vi "Dashboard Main.vi"() -> ()   [LabVIEW 2014]
uses:
  <vilib>/event_ctls.llb/eventvkey.ctl
  <vilib>/Rock Robotics/WPI/Dashboard/WPI_DashboardLogging Global.vi
  <vilib>/Rock Robotics/Network Tables/SD Read String Array.vi
  <vilib>/Rock Robotics/Network Tables/SD Read String.vi
  <vilib>/Utility/config.llb/Write Key (String).vi
  <vilib>/Utility/config.llb/Write Key (I32).vi
  <vilib>/Utility/cursorutil.llb/Set Cursor (Icon Pict).vi
  <vilib>/Utility/config.llb/NI_LVConfig.lvlib
panel:
  out "path":path
  in  "CameraView":bool
  in  "TCP":refnum<k5>
  in  "Rec Mode":enum32{"Stop", "Record", "Playback"}(radio)
  in  "Vision":u16(ring) items=["Camera Off", "USB Camera SW", "USB Camera HW", "IP Camera"]
  out "Camera IP":string
  out "Image Message":string="Timeout in Camera Communications"
  in  "Dashboard Tab":T1(tab)
  in  "Camera Settings":T2={"Frame Rate"=30, "Compression"=30, "Size"=1} {"Frame Rate" scale=1.0..30.0; "Size" items=["640x480", "320x240", "160x120"]}
  out "MotorChart R":cluster{"Numeric":dbl, "Numeric":dbl}(graph)
  out "MotorChart L":T3(graph)
  out "MotorSliders R":cluster{"MotorSlide1":dbl, "MotorSlide2":dbl} {"MotorSlide2" scale=-1.0..1.0 scale format="%#_2e"; "MotorSlide1" scale=-1.0..1.0 scale format="%#_2e"}
  out "MotorSliders L":T4 {"MotorSlide4 2" scale=0.0..14.0 scale format="%#_2e"; "MotorSlide2" scale=-1.0..1.0 scale format="%#_2e"; "MotorSlide1" scale=-1.0..1.0 scale format="%#_2e"}
  out "Gyro":dbl(knob) scale=0.0..360.0
  out "JS1 Z":dbl(slide) scale=-1.0..1.0 scale format="%#_2e"
  out "JS1 Graph":cluster{"X":dbl, "Y":dbl}[](graph)
  out "JS1 Buttons":T5
  out "JS2 Z":dbl(slide) scale=-1.0..1.0 scale format="%#_2e"
  out "JS2 Graph":cluster{"X":dbl, "Y":dbl}[](graph)
  out "JS2 Buttons":T5
  out "Mode":T6(ring)=enum."Auto Disabled"
  in  "DB Camera Config":bool
  out "fps":dbl format="%#.1g"
  out "Mbps":dbl format="%#.1g"
  out "Mbps 2":bool
  in  "DB/String 9":string
  in  "DB/String 8":string
  in  "DB/String 7":string
  in  "DB/String 6":string
  in  "DB/String 5":string
  in  "DB/String 4":string
  in  "DB/String 3":string
  in  "DB/String 2":string
  in  "DB/String 1":string
  in  "DB/String 0":string
  in  "DB/Slider 0":dbl(slide) scale=0.0..5.0
  in  "DB/Slider 1":dbl(slide) scale=0.0..5.0
  in  "DB/Slider 2":dbl(slide) scale=0.0..5.0
  in  "DB/Slider 3":dbl(slide) scale=0.0..5.0
  out "DB/LED 3":bool
  out "DB/LED 2":bool
  out "DB/LED 1":bool
  out "DB/LED 0":bool
  in  "DB/Button 3":bool
  in  "DB/Button 2":bool
  in  "DB/Button 1":bool
  in  "DB/Button 0":bool caption="New Name"
  out "Command":string
  in  "Enable Scripting":bool
  in  "Save":bool
  in  "Auton Edit Area":string
  in  "Edit":bool
  in  "Auton List":string(combo)
  out "CMD":string
  in  "Test Slider":dbl(slide) scale=0.0..100.0 scale format="%#_3g"
  in  "On/Off":bool caption="Solenoid"
  in  "Test Name":u16(ring) items=["Select the test to run...", "Example Test", "-------------------------------", "List of tests is built in robot code.", "Replace with your own automated tests."]
  in  "Test Tree":string(tree)
  in  "Motor":cluster{"Value":dbl, "Enable":bool} {"Value" scale=-1.0..1.0 scale format="%#_3g"}
  out "Progress":T7 {"Test Progress" scale=0.0..100.0}
  in  "Rev/Fwd":cluster{"Forward":bool, "Reverse":bool}
  in  "Test Ring":u16(ring) items=["Monochrome", "Color"]
  in  "Listbox":i32(listbox)
  out "Tree":string(tree)
  out "Camera Image":T8(plugin-control)
  out "Boolean":bool
  # "Left"
  # "Front"
  # "Right"
  # "Battery"
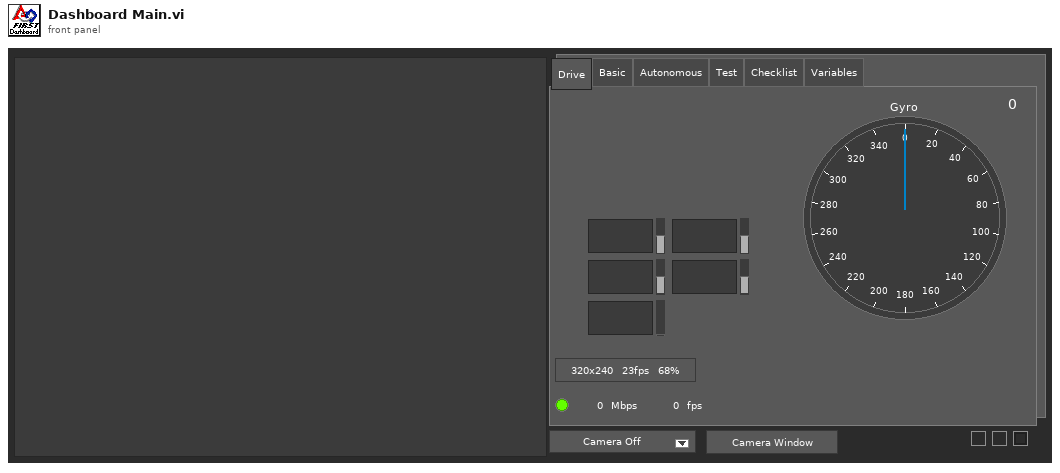
[diagram p1: front panel]
types:
  T1 = enum32{"Drive", "Basic", "Autonomous", "Test", "Checklist", "Variables"}
  T2 = cluster{"Frame Rate":i32, "Compression":i32, "Size":u16}
  T3 = cluster{"Numeric":dbl, "Numeric":dbl, "Battery V":dbl}
  T4 = cluster{"MotorSlide1":dbl, "MotorSlide2":dbl, "MotorSlide4 2":dbl}
  T5 = cluster{bool, bool, bool, bool, bool, bool, bool, bool, bool, bool, bool, bool}
  T6 = enum8{"Tele-Op Disabled", "Tele-Op Enabled", "Auto Disabled", "Auto Enabled", "Test Disabled", "Test Enabled", "Disconnected", "No Code", "E-Stop"}
  T7 = cluster{"Test Progress":u8, "Test Progress Text":string}
  T8 = typedef "IMAQ Image.ctl" = refnum<image>
  T9 = enum32{"Drive", "Basic", "Custom", "Test", "Checklist", "Variables"}
  T10 = typedef "Image Type" = u32
  T11 = cluster{"Camera Image":refnum<vi>, "Dashboard Tab":refnum<vi>, "Boolean":refnum<vi>, "Vision":refnum<vi>, "Rec Mode":refnum<vi>, "Test Slider":refnum<vi>, "On/Off ":refnum<vi>, "Test Ring":refnum<vi>, "Rev/Fwd":refnum<vi>, "Test Name":refnum<vi>, "Motor":refnum<vi>, "Progress":refnum<vi>, "CheckList":refnum<vi>, "Tree":refnum<vi>, "Test Tree":refnum<vi>}
  T12 = cluster{"Error Strings":string, "Disable Counts":cluster{u16, u16}, "Rail Faults":cluster{u16, u16, u16}, "Robot IP":string, "DB Mode":u8, "Event Info":cluster{"Name":string, "Type":u8, "Number":u16, "Replay":u8}, "Camera Addr":string}
  T13 = cluster{"Storage":cluster{"Disk Free":u64, "RAM Block":u32, "RAM free":u32}, "CPU Utilization":cluster{"CPU % ISR":sgl, "CPU % Time Crit":sgl, "CPU % Timed Str":sgl, "CPU % High":sgl, "CPU % Above":sgl, "CPU % Normal":sgl, "CPU % Low":sgl}, "CAN":cluster{"% Bus Utilization":sgl, "Bus Off Cnt":u32, "TX_FIFO Full Cnt":u32, "Receive Error Cnt":u8, "Transmit Error Cnt":u8}, "HID":cluster{"HID Outputs":u32, "Rumble Low":u16, "Rumble High":u16}[]}
  T14 = cluster{"Status bits":cluster{"Test Mode":bool, "Autonomous":bool, "Enabled":bool, "Code Start":bool, "Brownout":bool, "Reserved 2":bool, "Reserved 3":bool, "E-Stop":bool}, "Code Trace":cluster{"Disabled":bool, "TeleOp":bool, "Auto":bool, "Test":bool}, "Controller Type":enum16{"unknown", "cRIO", "roboRio"}, "Code?":enum16{"unknown", "noCode", "code"}, "Battery V":dbl}
  T15 = cluster{"Control Bits":cluster{"TestMode":bool, "Autonomous":bool, "Enabled":bool, "FMS Present":bool, bool, bool, bool, "E-Stop":bool}, "Team Station ":u8, "Countdown":sgl, "Joystick Values":cluster{"Axes":dbl[], "Buttons":bool[], "POVs":i16[]}[]}
  T16 = cluster{"Axes":dbl[], "Buttons":bool[], "POVs":i16[]}[]
  T17 = cluster{"Axes":dbl[], "Buttons":bool[], "POVs":i16[]}
  T18 = cluster{"Buttons[0]":bool, "Buttons[1]":bool, "Buttons[2]":bool, "Buttons[3]":bool, "Buttons[4]":bool, "Buttons[5]":bool, "Buttons[6]":bool, "Buttons[7]":bool, "Buttons[8]":bool, "Buttons[9]":bool, "Buttons[10]":bool, "Buttons[11]":bool}
  T19 = typedef "NI_LVConfig.lvlib/Config Data RefNum.ctl" = refnum<k1>
  T20 = cluster{"Operation":enum16{"Update", "Clear"}, "Color Box":u32}[]
  T21 = typedef "eventvkey.ctl" = enum16{"ASCII", "Enter", "Return", "Shift", "Ctrl", "Alt", "Cmd", "Opt", "Caps", "NumLock", "Clear", "Break", "Up", "Down", "Left", "Right", "Insert", "Delete", "Home", "End", "PageUp", "PageDown", "Escape", "Help", "Pause", "ScrollLock", "F1", "F2", "F3", "F4", "F5", "F6", "F7", "F8", "F9", "F10", "F11", "F12", "F13", "F14", "F15", "F16", "F17", "F18", "F19", "F20", "F21", "F22", "F23", "F24", "Play", "VolumeUp", "VolumeDown", "Mute", "Two Byte Char"}
  T22 = cluster{"Image Size":bool, "Image Type":bool, "Pixel Value":bool, "ROI Information":bool, "Zoom Factor":bool}
  T23 = enum8{"Enabled", "Disabled", "Disabled and Grayed Out"}
  T24 = enum16{"open", "replace", "create", "open or create", "replace or create", "replace or create with confirmation"}
  T25 = cluster{"Operation":enum16{"Update", "Clear"}, "Color Box":u32}
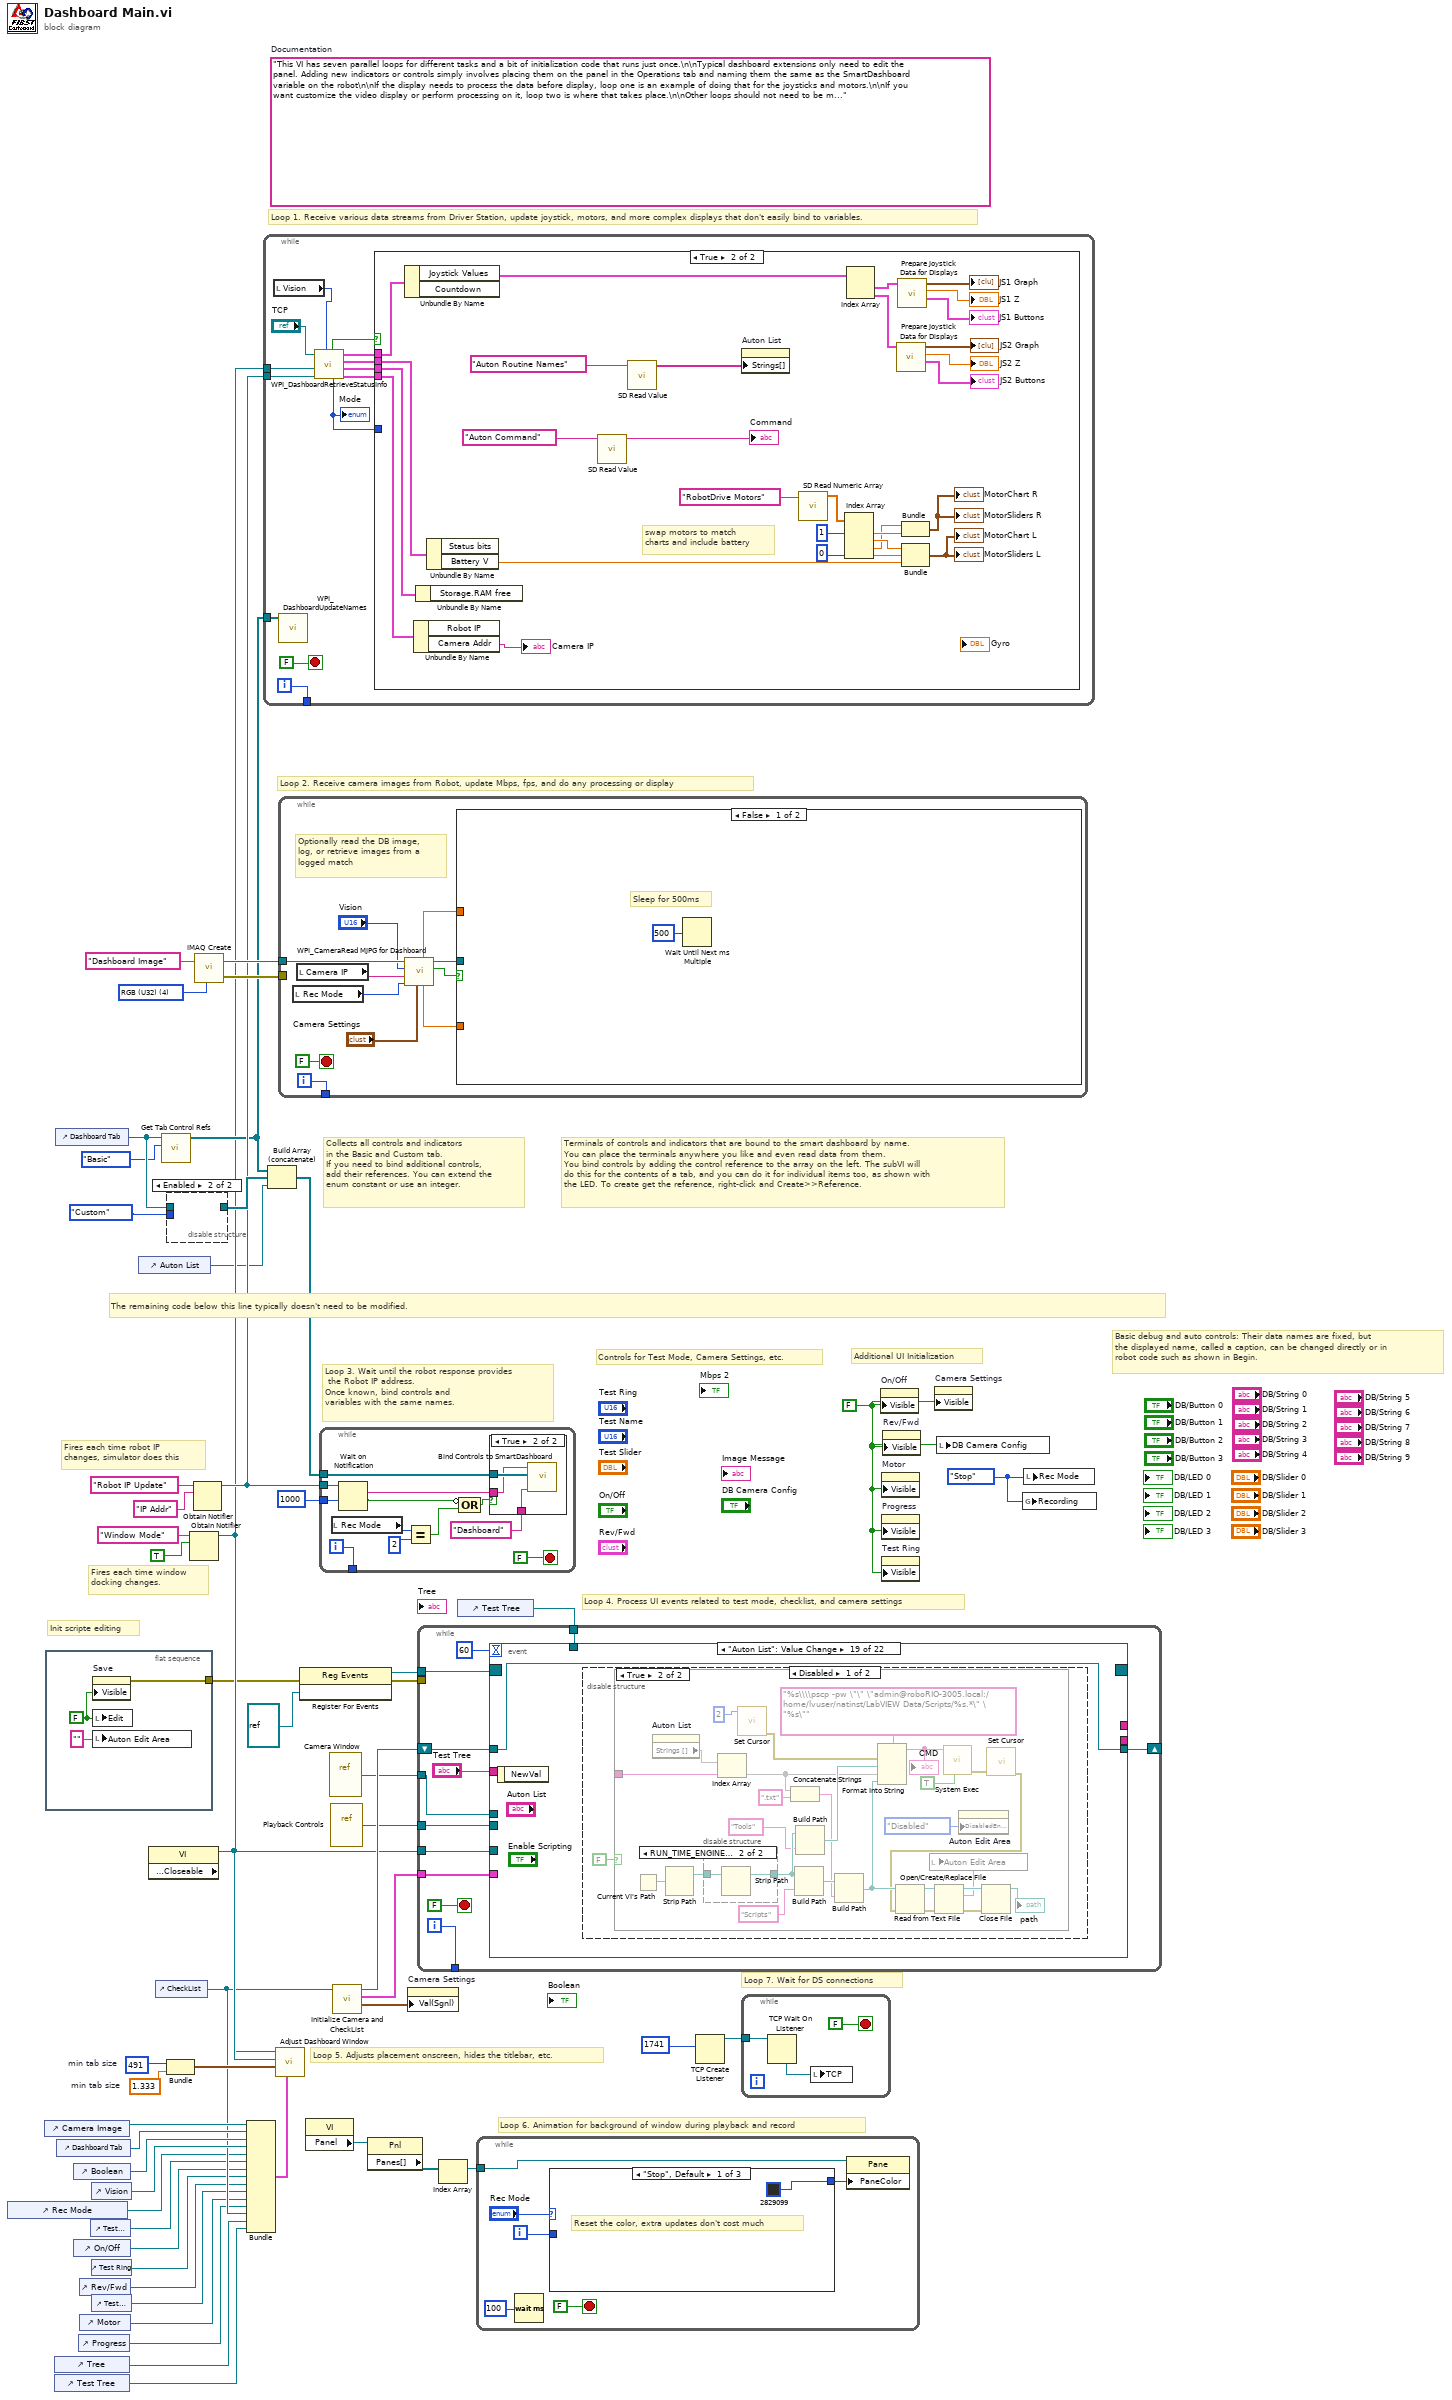
[diagram p0: block diagram]
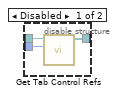
[diagram p2: hidden frame]
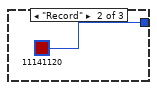
[diagram p4: hidden frame]
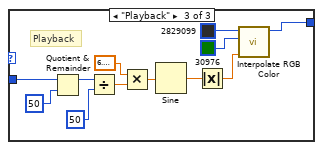
[diagram p5: hidden frame]
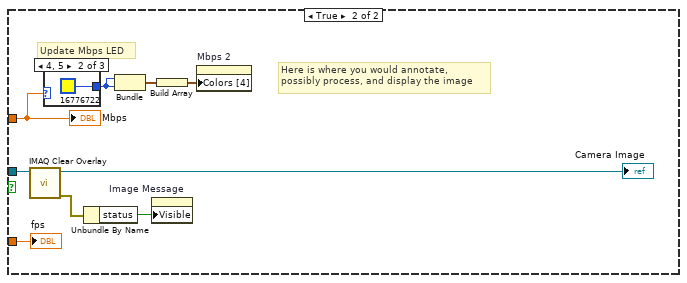
[diagram p7: hidden frame]
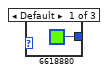
[diagram p8: hidden frame]
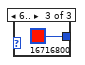
[diagram p9: hidden frame]
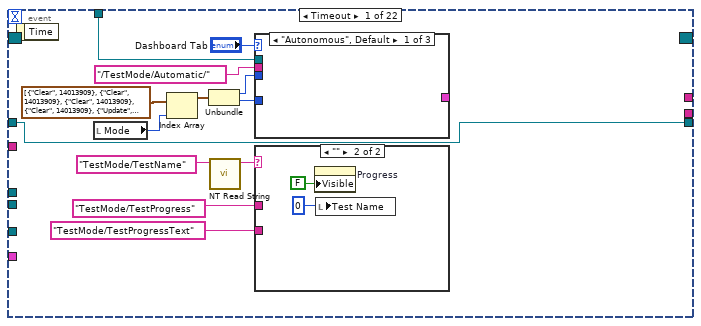
[diagram p10: hidden frame]
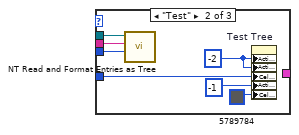
[diagram p11: hidden frame]
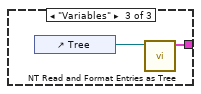
[diagram p12: hidden frame]
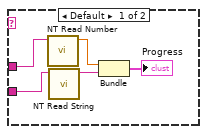
[diagram p13: hidden frame]
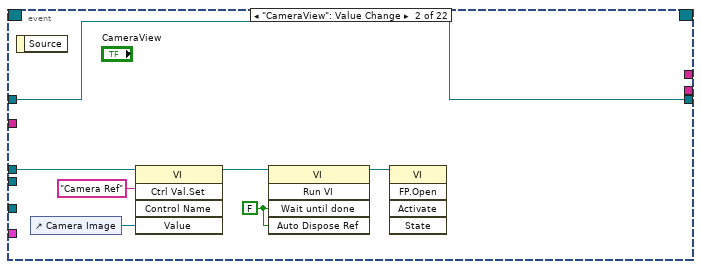
[diagram p14: hidden frame]
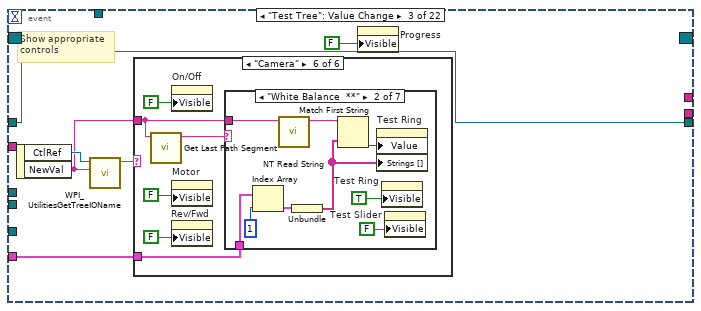
[diagram p15: hidden frame]
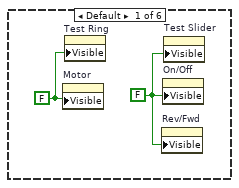
[diagram p16: hidden frame]
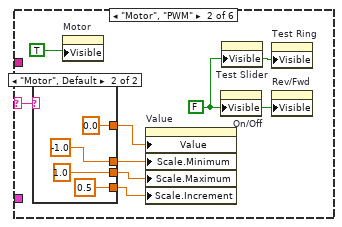
[diagram p17: hidden frame]
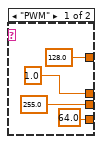
[diagram p18: hidden frame]
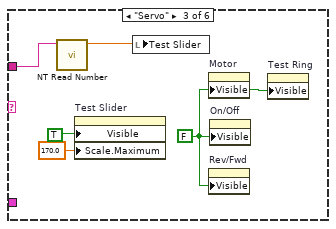
[diagram p19: hidden frame]
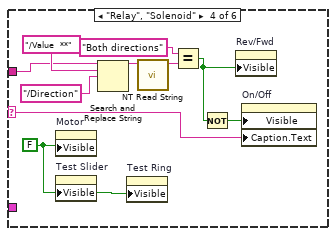
[diagram p20: hidden frame]
diagram:
  w27 = 491  # min tab size
  w26 = 1.333  # min tab size
  w35 = enum32{"Stop", "Record", "Playback"}."Stop" ("Rec Mode")
  w9 = FALSE ("Visible")
  (unwired) "This VI has seven parallel loops for different tasks and a bit of initialization code that runs just once.\n\nTypical dashboard extensions only need to edit the panel. Adding new indicators or controls simply involves placing them on the panel in the Operations tab and naming them the same as the SmartDashboard variable on the robot\n\nIf the display needs to process the data before display, loop one is an example of doing that for the joysticks and motors.\n\nIf you want customize the video display or perform processing on it, loop two is where that takes place.\n\nOther loops should not need to be modified. They are pretty standard, and document the task they perform."  # Documentation
  w55 = T10 4 items=["Grayscale (U8)", "Grayscale (I16)", "Grayscale (SGL)", "Complex (CSG)", "RGB (U32)", "HSL (U32)", "RGB (U64)"] ("Image Type")
  # "Init scripte editing"
  # "Loop 7. Wait for DS connections"
  # "Basic debug and auto controls: Their data names are fixed, but\nthe displayed name, called a caption, can be changed directly or in\nrobot code such as shown in Begin."
  # "Controls for Test Mode, Camera Settings, etc."
  # "Additional UI Initialization"
  # "Loop 6. Animation for background of window during playback and record"
  # "Fires each time robot IP\nchanges, simulator does this"
  # "Fires each time window\ndocking changes."
  # "Collects all controls and indicators\nin the Basic and Custom tab.\nIf you need to bind additional controls,\nadd their references. You can extend the\nenum constant or use an integer."
  # "The remaining code below this line typically doesn't need to be modified."
  # "Loop 4. Process UI events related to test mode, checklist, and camera settings"
  # "Terminals of controls and indicators that are bound to the smart dashboard by name.\nYou can place the terminals anywhere you like and even read data from them.\nYou bind controls by adding the control reference to the array on the left. The subVI will\ndo this for the contents of a tab, and you can do it for individual items too, as shown with\nthe LED. To create get the reference, right-click and Create>>Reference."
  # "Loop 3. Wait until the robot response provides\n the Robot IP address.\nOnce known, bind controls and\nvariables with the same names."
  # "Loop 5. Adjusts placement onscreen, hides the titlebar, etc."
  # "Loop 1. Receive various data streams from Driver Station, update joystick, motors, and more complex displays that don't easily bind to variables."
  # "Loop 2. Receive camera images from Robot, update Mbps, fps, and do any processing or display"
  n1 = control-ref of="Rec Mode"() -> (w15:refnum<vi>)
  n2 = control-ref of="Camera Image"() -> (w30:refnum<vi>)
  n3 = flat-sequence {
    tunnel: [w56] -> w1
    frame #0 {
      w57 = FALSE ("Edit")
      n4 = property on="Save" class="Bool"("Visible"=w57) -> (error out=w56:errorcluster)  [unwired: 2 in, 1 out]
      n5 = local write "Edit"(w57) -> ()
      n6 = local write "Auton Edit Area"("" ("Auton Edit Area")) -> ()
    }
  }
  n7 = control-ref of="Tree"() -> (w19:refnum<vi>)
  n8 = control-ref of="Test Tree"() -> (w18:refnum<vi>)
  n9 = control-ref of="Dashboard Tab"() -> (w33:refnum<vi>)
  n10 = control-ref of="Dashboard Tab"() -> (w29:refnum<vi>)
  n11 = control-ref of="Boolean"() -> (w24:refnum<vi>)
  n12 = control-ref of="On/Off"() -> (w13:refnum<vi>)
  n13 = control-ref of="Progress"() -> (w10:refnum<vi>)
  n14 = control-ref of="Rev/Fwd"() -> (w11:refnum<vi>)
  n15 = control-ref of="Motor"() -> (w16:refnum<vi>)
  n16 = control-ref of="Test Slider"() -> (w14:refnum<vi>)
  n17 = control-ref of="Vision"() -> (w28:refnum<vi>)
  n18 = control-ref of="Test Ring"() -> (w12:refnum<vi>)
  n19 = control-ref of="Test Name"() -> (w17:refnum<vi>)
  n20 = control-ref of="Auton List"() -> (w2:refnum<vi>)
  n21 = property class="VI" props=["Front Panel.Closeable"]() -> (reference out=w34:refnum<vi>)  [unwired: 2 in, 2 out]
  n22 = control-ref of="CheckList"() -> (w20:refnum<vi>)
  n23 = call <vilib>:"Get Tab Control Refs.vi"("Page Index"=T9."Basic" ("Dashboard Tab"), "TabControl in"=w33) -> ("ControlsOnPage"=w7:refnum<vi>[])  [unwired: 9 in]
  n24 = disable-structure shown="Enabled" {
    disable-tunnel: w33 -> [w61 _]
    disable-tunnel: [w60 _] -> w32
    disable-tunnel: T9."Custom" ("Dashboard Tab") -> [w59 _]
    frame Disabled {
      n25 = call <vilib>:"Get Tab Control Refs.vi"("Page Index"=w59, "TabControl in"=w61) -> ("ControlsOnPage"=w60:refnum<vi>[])  [unwired: 9 in]
    }
    frame Enabled {
    }
  }
  n26 = Bundle("min tab size"=w27, "min tab size"=w26) -> (w25:cluster{"min tab size":i32, "min tab size":dbl})  [unwired: 1 in]
  n27 = Obtain Notifier(name (unnamed)="Window Mode", notification data type=TRUE) -> (notifier out=w6:refnum<notifier>)  [unwired: 2 in, 2 out]
  n28 = Obtain Notifier(name (unnamed)="Robot IP Update", notification data type="IP Addr" ("name (unnamed)")) -> (notifier out=w8:refnum<notifier>)  [unwired: 2 in, 2 out]
  n29 = call "IMAQ Create"("Image Name"="Dashboard Image", "Image Type"=w55) -> ("New Image"=w53:T8, "error out"=w52:errorcluster)  [unwired: 2 in, 1 out]
  n30 = Bundle("Camera Image"=w30, "Dashboard Tab"=w29, "Boolean"=w24, "Vision"=w28, "Rec Mode"=w15, "Test Slider"=w14, "On/Off"=w13, "Test Ring"=w12, "Rev/Fwd"=w11, "Test Name"=w17, "Motor"=w16, "Progress"=w10, "CheckList"=w20, "Tree"=w19, "Test Tree"=w18) -> (w21:T11)  [unwired: 1 in]
  n31 = while {
    tunnel: [w73] -> _
    tunnel: w8 -> [w67]
    tunnel: w7 -> [w66]
    tunnel: w6 -> [w62]
    i -> [w73]
    stop <- FALSE stop-if-true
    n32 = local read "Vision"() -> (w64:u16)
    n33 = call <vilib>:"WPI_DashboardUpdateNames.vi"("Controls on Tab"=w66) -> ()  [unwired: 11 in]
    n34 = call <vilib>:"WPI_DashboardRetrieveStatusInfo.vi"("Vision"=w64, "Binding Refnum"=w67, "Window Mode Notifier"=w62, "TCP Cnx"="TCP") -> ("Power and Errors"=w68:T12, "Robot Metrics"=w71:T13, "Status Info"=w72:T14, "Control Info"=w69:T15, "Robot Mode"=w65:T6, "Process?"=w70:bool)  [unwired: 2 in]
    "Mode" <- w65
    n35 = case shown="True" w70 {
      tunnel: w72 -> [_ w103]
      tunnel: w71 -> [_ w102]
      tunnel: w69 -> [_ w101]
      tunnel: w68 -> [_ w100]
      tunnel: w65 -> [_ _]
      frame False {
      }
      frame True {
        # "swap motors to match\ncharts and include battery"
        n36 = Unbundle By Name(w101) -> ("Joystick Values"=w88:T16)  [unwired: 1 out]
        n37 = Unbundle By Name(w100) -> ("Camera Addr"=→"Camera IP":string)  [unwired: 1 out]
        n38 = Unbundle By Name(w102) -> ()  [unwired: 1 out]
        n39 = Unbundle By Name(w103) -> ("Battery V"=w89:dbl)  [unwired: 1 out]
        n40 = call-poly <vilib>:"SD Read Value.vi"("Name"="Auton Command") -> ("String"=→"Command":string)  [unwired: 8 in, 2 out]
        n41 = call-poly <vilib>:"SD Read Value.vi"("Name"="Auton Routine Names") -> ("String Array"=w78:string[])  [unwired: 9 in, 1 out]
        n42 = property on="Auton List" class="CmbBox"("Strings[]"=w78) -> ()  [unwired: 2 in, 2 out]
        n43 = call <vilib>:"SD Read Numeric Array.vi"("Name"="RobotDrive Motors") -> ("Numeric Array"=w91:dbl[])  [unwired: 8 in, 2 out]
        n44 = Index Array(array=w91, index #1=1, index #4=0) -> (element #1=w95:dbl, element #2=w96:dbl, element #3=w94:dbl, element #4=w99:dbl)  [unwired: 2 in]
        n45 = Index Array(array=w88) -> (element #1=w87:T17, element #2=w82:T17)  [unwired: 2 in]
        n46 = call "Prepare Joystick Data for Displays.vi"("Joystick Values"=w82) -> ("Buttons"=→"JS2 Buttons":T18, "Z Axis"=→"JS2 Z":dbl, "Cartesian Data"=→"JS2 Graph":cluster{"X axis":dbl, "X axis":dbl}[])  [unwired: 8 in]
        n47 = call "Prepare Joystick Data for Displays.vi"("Joystick Values"=w87) -> ("Buttons"=→"JS1 Buttons":T18, "Z Axis"=→"JS1 Z":dbl, "Cartesian Data"=→"JS1 Graph":cluster{"X axis":dbl, "X axis":dbl}[])  [unwired: 8 in]
        n48 = Bundle("Numeric"=w94, "Numeric"=w95) -> (→"MotorChart R" →"MotorSliders R":cluster{"Numeric":dbl, "Numeric":dbl})  [unwired: 1 in]
        n49 = Bundle("Numeric"=w96, "Numeric"=w99, "Battery V"=w89) -> (→"MotorChart L" →"MotorSliders L":T3)  [unwired: 1 in]
      }
    }
  }
  n50 = Build Array (concatenate)(w7, w32, w2) -> (w31:refnum<vi>[])
  n51 = call "Adjust Dashboard Window.vi"("Sizing Refnums"=w21, "Size Constraints"=w25, "VI"=w34, "Notifier in"=w6) -> ()  [unwired: 8 in]
  n52 = while {
    tunnel: w53 -> [w112]
    tunnel: w52 -> [_]
    tunnel: [w113] -> _
    i -> [w113]
    stop <- FALSE stop-if-true
    # "Optionally read the DB image,\nlog, or retrieve images from a\nlogged match"
    n53 = local read "Rec Mode"() -> (w106:enum32{"Stop", "Record", "Playback"})
    n54 = local read "Camera IP"() -> (w104:string)
    n55 = call <vilib>:"WPI_CameraRead MJPG for Dashboard.vi"("Camera Settings"="Camera Settings", "Rec Mode"=w106, "Camera IP"=w104, "Camera Mode"="Vision", "Refnum in"=w112) -> ("Active"=w110:bool, "Refnum out"=w111:T8, "FPS"=w109:dbl, "Bandwidth (Mbps)"=w108:dbl)  [unwired: 3 in]
    n56 = case shown="False" w110 {
      tunnel: w111 -> [_ w119]
      tunnel: w108 -> [_ w118]
      tunnel: w109 -> [_ w116]
      frame False {
        # "Sleep for 500ms"
        n57 = Wait Until Next ms Multiple(millisecond multiple=u32 500) -> ()  [unwired: 1 out]
      }
      frame True {
        # "Here is where you would annotate,\npossibly process, and display the image"
        # "Update Mbps LED"
        n58 = call "IMAQ Clear Overlay"("Image"=w119) -> ("error out"=w123:errorcluster, "Image Out"=→"Camera Image":T8)  [unwired: 2 in, 7 out]
        n59 = case shown="4, 5" w118 {
          tunnel: [u32 6618880 ("Color Box") u32 16776722 ("Color Box") u32 16716800 ("Color Box")] -> w120
          frame Default {
          }
          frame 4, 5 {
          }
          frame 6.. {
          }
        }
        n60 = Unbundle By Name(w123) -> ("status"=w124:bool)
        n61 = Bundle("Color Box"=w120, "Color Box"=w120) -> (w122:cluster{"Color Box":u32, "Color Box":u32})  [unwired: 1 out]
        n62 = property on="Image Message" class="Str"("Visible"=w124) -> ()  [unwired: 2 in, 2 out]
        n63 = Build Array(w122) -> (w121:cluster{"Color Box":u32, "Color Box":u32}[])
        n64 = property on="Mbps 2" class="Bool (strict)"("Colors [4]"=w121) -> ()  [unwired: 2 in, 2 out]
        "Mbps" <- w118
        "fps" <- w116
      }
    }
  }
  n65 = register-events(error in=w1, refnum<vi> refnum) -> (reference out=w39:refnum<event-registration>, error out=w38:errorcluster)  [unwired: 1 in]
  n66 = property class="VI"() -> ("Panel"=w42:refnum<vi>)  [unwired: 2 in, 2 out]
  n67 = while {
    tunnel: w31 -> [w139]
    tunnel: w8 -> [w137]
    tunnel: [w135] -> _
    tunnel: u32 1000 ("milliseconds to wait") -> [w134]
    i -> [w135]
    stop <- FALSE stop-if-true
    n68 = local read "Rec Mode"() -> (w130:enum32{"Stop", "Record", "Playback"})
    n69 = Wait on Notification(notifier=w137, timeout in ms (-1)=w134) -> (notification=w136:string, timed out?=w132:bool)  [unwired: 2 in, 2 out]
    n70 = Equal?(x=w130, y=u16 2 ("Rec Mode")) -> (x = y?=w131:bool)
    n71 = Compound Arithmetic op=OR(invert w132, w131) -> (w133:bool)
    n72 = case shown="True" w133 {
      tunnel: w139 -> [_ w142]
      tunnel: w136 -> [_ w141]
      tunnel: "Dashboard" -> [_ w140]
      frame False {
      }
      frame True {
        n73 = call <vilib>:"Bind Controls to SmartDashboard.vi"("Client Name"=w140, "Bound Control Refs"=w142, "Server IP Address"=w141) -> ()  [unwired: 9 in]
      }
    }
  }
  n74 = vi-ref "Camera Window.vi"() -> (w3:refnum<vi>)
  n75 = vi-ref "Playback Controls.vi"() -> (w40:refnum<vi>)
  n76 = call "Initialize Camera and CheckList.vi"("ListBox in"=w20) -> ("Cluster"=w46:cluster{"value":i32, "value":i32, "index":i32}, "Array"=w47:cluster{string[]}[], "File Refnum"=w45:T19)  [unwired: 8 in]
  n77 = property class="Pnl"(reference=w42) -> ("Panes[]"=w43:refnum<vi>[])  [unwired: 1 in, 2 out]
  n78 = property on="Camera Settings" class="Clust (strict)"("Val(Sgnl)"=w46) -> ()  [unwired: 2 in, 2 out]
  n79 = Index Array(array=w43) -> (element=w41:refnum<vi>)  [unwired: 1 in]
  n80 = control-ref of="Test Tree"() -> (w44:refnum<vi>)
  n81 = while {
    tunnel: w47 -> [w151]
    shift-right: [w150] -> _
    shift-left: w45 -> [w149]
    tunnel: [w148] -> _
    tunnel: w44 -> [w147]
    tunnel: w40 -> [w146]
    tunnel: w39 -> [w145]
    tunnel: w38 -> [_]
    tunnel: w34 -> [w144]
    tunnel: w3 -> [w143]
    i -> [w148]
    stop <- FALSE stop-if-true
    n82 = event shown="[18] \"Auton List\": Value Change" {
      selector: w145 -> [_ _ _ _ _ _ _ _ _ _ _ _ _ _ _ _ _ _ _ _ _ _]
      dyn-events: [_ _ _ _ _ _ _ _ _ _ _ _ _ _ w396 _ _ _ _ _ _ _] -> _
      timeout: u32 60 ("milliseconds to wait") -> [_ _ _ _ _ _ _ _ _ _ _ _ _ _ _ _ _ _ _ _ _ _]
      tunnel: w147 -> [w163 _ _ _ _ _ _ _ _ _ _ _ _ _ _ _ _ _ _ _ _ _]
      tunnel: "Test Tree" -> [_ _ _ _ _ _ _ _ _ w365 w373 w375 w379 w387 _ _ _ _ _ _ _ _]
      tunnel: w151 -> [_ _ w192 _ _ _ _ w329 w359 _ _ _ _ _ _ _ _ _ _ _ _ _]
      tunnel: [w159 w190 w191 w290 w295 w303 w315 w328 w352 w364 w371 w374 w378 w386 w398 w412 w416 w428 w429 w462 w486 w492] -> w150
      tunnel: w149 -> [w159 w190 w191 w290 w295 w303 w315 w327 w352 w364 w371 w374 w378 w386 w398 w412 w416 w428 w429 w462 w486 w492]
      tunnel: w146 -> [_ _ _ _ _ _ _ _ _ _ _ _ _ _ w399 _ w419 _ _ _ _ _]
      tunnel: w144 -> [_ _ _ _ _ _ _ _ _ _ _ _ _ _ w394 _ _ _ _ _ _ _]
      tunnel: w143 -> [_ w189 _ _ _ _ _ _ _ _ _ _ _ _ _ _ w413 _ _ _ _ _]
      tunnel: [_ _ _ _ _ _ _ _ _ _ _ _ _ _ _ _ _ _ _ _ w464 _] -> _
      tunnel: [_ _ _ _ _ _ _ _ _ _ _ _ _ _ _ _ _ _ _ _ w463 _] -> _
      event Timeout {
        n83 = event-data() -> ()  [unwired: 1 in, 1 out]
        n84 = local read "Mode"() -> (w162:T6)
        n85 = Index Array(array=T20 [{"Operation"=enum."Clear", "Color Box"=14013909}, {"Operation"=enum."Clear", "Color Box"=14013909}, {"Operation"=enum."Clear", "Color Box"=14013909}, {"Operation"=enum."Clear", "Color Box"=14013909}, {"Operation"=enum."Update", "Color Box"=14013909}, {"Operation"=enum."Update", "Color Box"=16777215}, {"Operation"=enum."Clear", "Color Box"=14013909}, {"Operation"=enum."Clear", "Color Box"=14013909}, {"Operation"=enum."Clear", "Color Box"=14013909}], index=w162) -> (element=w157:T25)
        n86 = Unbundle(w157) -> ("Operation"=w156:enum16{"Update", "Clear"}, "Color Box"=w155:u32)
        n87 = call <vilib>:"NT Read String.vi"("Name"="TestMode/TestName") -> ("String"=w166:string)  [unwired: 9 in, 1 out]
        n88 = case shown="\"Autonomous\", Default" "Dashboard Tab" {
          tunnel: w163 -> [_ w174 _]
          tunnel: "/TestMode/Automatic/" ("Name Pattern") -> [_ w173 _]
          tunnel: w156 -> [_ w172 _]
          tunnel: [_ _ w176] -> _
          tunnel: w155 -> [_ w168 _]
          frame "Autonomous", Default {
          }
          frame "Test" {
            w171 = -2 ("Active Item:Row Number")
            n89 = call <vilib>:"NT Read and Format Entries as Tree.vi"("Operation"=w172, "Name Pattern"=w173, "Tree Refnum"=w174) -> ()  [unwired: 7 in, 2 out]
            n90 = property on="Test Tree" class="Tree (strict)"("Active Item Row Number"=w171, "ActiveColNum"=w171, "CellBG"=w168, "Active Item Row Number"=-1 ("Active Item:Row Number"), "CellBG"=u32 5789784 ("Color Box")) -> ()  [unwired: 2 in, 2 out]
          }
          frame "Variables" {
            n91 = control-ref of="Tree"() -> (w175:refnum<vi>)
            n92 = call <vilib>:"NT Read and Format Entries as Tree.vi"("Tree Refnum"=w175) -> ("Formatted Strings"=w176:cluster{"Name":string, "Value":string}[])  [unwired: 9 in, 1 out]
          }
        }
        n93 = case shown="\"\"" w166 {
          tunnel: "TestMode/TestProgress" ("Name") -> [w178 _]
          tunnel: "TestMode/TestProgressText" ("Name") -> [w177 _]
          frame Default {
            n94 = call <vilib>:"NT Read Number.vi"("Name"=w178) -> ("Numeric"=w179:dbl)  [unwired: 9 in, 1 out]
            n95 = call <vilib>:"NT Read String.vi"("Name"=w177) -> ("String"=w180:string)  [unwired: 9 in, 1 out]
            n96 = Bundle("Numeric"=w179, "String"=w180) -> (→"Progress":cluster{"Numeric":dbl, "String":string})  [unwired: 1 in]
          }
          frame "" {
            n97 = property on="Progress" class="Clust (strict)"("Visible"=FALSE) -> ()  [unwired: 2 in, 2 out]
            n98 = local write "Test Name"(u16 0) -> ()
          }
        }
      }
      event "CameraView": Value Change {
        w188 = FALSE ("Wait Until Done")
        n99 = event-data() -> ()  [unwired: 1 in, 1 out]
        n100 = control-ref of="Camera Image"() -> (w185:refnum<vi>)
        n101 = invoke class="VI" method="Ctrl Val.Set"(reference=w189, "Control Name"="Camera Ref", "Value"=w185) -> (reference out=w186:refnum<vi>)  [unwired: 2 in, 4 out]
        n102 = invoke class="VI" method="Run VI"(reference=w186, "Wait until done"=w188, "Auto Dispose Ref"=w188) -> (reference out=w187:refnum<vi>)  [unwired: 2 in, 4 out]
        n103 = invoke class="VI" method="FP.Open"(reference=w187) -> ()  [unwired: 4 in, 5 out]
      }
      event "Test Tree": Value Change {
        # "Show appropriate\ncontrols"
        n104 = event-data() -> ("CtlRef"=w195:refnum<vi>, "NewVal"=w193:string)  [unwired: 1 in]
        n105 = call <vilib>:"WPI_UtilitiesGetTreeIOName.vi"("NewVal"=w193, "TreeControl in"=w195) -> ("I/O Name"=w196:string)  [unwired: 9 in]
        n106 = case shown="\"Camera\"" w196 {
          selector: w196 -> [_ w203 _ w221 w230 _]
          tunnel: w193 -> [_ _ w218 w220 _ w237]
          tunnel: w192 -> [_ _ _ _ _ w236]
          frame Default {
            w198 = FALSE ("Visible")
            w197 = FALSE ("Visible")
            n107 = property on="Motor" class="Clust (strict)"("Visible"=w197) -> ()  [unwired: 2 in, 2 out]
            n108 = property on="Test Ring" class="Ring (strict)"("Visible"=w197) -> ()  [unwired: 2 in, 2 out]
            n109 = property on="Rev/Fwd" class="Clust (strict)"("Visible"=w198) -> ()  [unwired: 2 in, 2 out]
            n110 = property on="On/Off" class="Bool (strict)"("Visible"=w198) -> ()  [unwired: 2 in, 2 out]
            n111 = property on="Test Slider" class="Slide (strict)"("Visible"=w198) -> ()  [unwired: 2 in, 2 out]
          }
          frame "Motor", "PWM" {
            w204 = FALSE ("Visible")
            n112 = case shown="\"Motor\", Default" w203 {
              tunnel: [1.0 ("Value") -1.0 ("Value")] -> w202
              tunnel: [255.0 ("Value") 1.0 ("Value")] -> w201
              tunnel: [128.0 ("Value") 0.0 ("Value")] -> w200
              tunnel: [64.0 ("Value") 0.5 ("Value")] -> w199
              frame "PWM" {
              }
              frame "Motor", Default {
              }
            }
            n113 = property on="Motor" class="Clust (strict)"("Visible"=TRUE) -> ()  [unwired: 2 in, 2 out]
            n114 = property on="Value" class="Slide (strict)"("Value"=w200, "Scale.Minimum"=w202, "Scale.Maximum"=w201, "Scale.Increment"=w199) -> ()  [unwired: 2 in, 2 out]
            n115 = property on="On/Off" class="Bool (strict)"("Visible"=w204) -> ()  [unwired: 2 in, 2 out]
            n116 = property on="Test Slider" class="Slide (strict)"("Visible"=w204) -> ()  [unwired: 2 in, 2 out]
            n117 = property on="Test Ring" class="Ring (strict)"("Visible"=w204) -> ()  [unwired: 2 in, 2 out]
            n118 = property on="Rev/Fwd" class="Clust (strict)"("Visible"=w204) -> ()  [unwired: 2 in, 2 out]
          }
          frame "Servo" {
            w216 = FALSE ("Visible")
            n119 = call <vilib>:"NT Read Number.vi"("Name"=w218) -> ("Numeric"=w217:dbl)  [unwired: 9 in, 1 out]
            n120 = property on="Test Slider" class="Slide (strict)"("Visible"=TRUE, "Scale.Maximum"=170.0 ("Scale.Range:Maximum")) -> ()  [unwired: 2 in, 2 out]
            n121 = local write "Test Slider"(w217) -> ()
            n122 = property on="Motor" class="Clust (strict)"("Visible"=w216) -> ()  [unwired: 2 in, 2 out]
            n123 = property on="Rev/Fwd" class="Clust (strict)"("Visible"=w216) -> ()  [unwired: 2 in, 2 out]
            n124 = property on="On/Off" class="Bool (strict)"("Visible"=w216) -> ()  [unwired: 2 in, 2 out]
            n125 = property on="Test Ring" class="Ring (strict)"("Visible"=w216) -> ()  [unwired: 2 in, 2 out]
          }
          frame "Relay", "Solenoid" {
            w219 = FALSE ("Visible")
            n126 = property on="Motor" class="Clust (strict)"("Visible"=w219) -> ()  [unwired: 2 in, 2 out]
            n127 = property on="Test Slider" class="Slide (strict)"("Visible"=w219) -> ()  [unwired: 2 in, 2 out]
            n128 = Search and Replace String(input string=w220, search string="/Value  **", replace string="/Direction") -> (result string=w226:string)  [unwired: 5 in, 3 out]
            n129 = property on="Test Ring" class="Ring (strict)"("Visible"=w219) -> ()  [unwired: 2 in, 2 out]
            n130 = call <vilib>:"NT Read String.vi"("Name"=w226) -> ("String"=w224:string)  [unwired: 9 in, 1 out]
            n131 = Equal?(x="Both directions", y=w224) -> (x = y?=w222:bool)
            n132 = Not(x=w222) -> (.not. x?=w223:bool)
            n133 = property on="Rev/Fwd" class="Clust (strict)"("Visible"=w222) -> ()  [unwired: 2 in, 2 out]
            n134 = property on="On/Off" class="Bool (strict)"("Visible"=w223, "Caption.Text"=w221) -> ()  [unwired: 2 in, 2 out]
          }
          frame "Compressor", "Digital Out" {
            w229 = FALSE ("Visible")
            # "Get direction and finish"
            n135 = property on="Motor" class="Clust (strict)"("Visible"=w229) -> ()  [unwired: 2 in, 2 out]
            n136 = property on="Test Slider" class="Slide (strict)"("Visible"=w229) -> ()  [unwired: 2 in, 2 out]
            n137 = property on="Test Ring" class="Ring (strict)"("Visible"=w229) -> ()  [unwired: 2 in, 2 out]
            n138 = property on="On/Off" class="Bool (strict)"("Visible"=TRUE, "Caption.Text"=w230) -> ()  [unwired: 2 in, 2 out]
            n139 = property on="Rev/Fwd" class="Clust (strict)"("Visible"=FALSE) -> ()  [unwired: 2 in, 2 out]
          }
          frame "Camera" {
            n140 = call <vilib>:"Get Last Path Segment.vi"("String in"=w237) -> ("String out"=w238:string)  [unwired: 10 in]
            n141 = property on="On/Off" class="Bool (strict)"("Visible"=FALSE) -> ()  [unwired: 2 in, 2 out]
            n142 = property on="Motor" class="Clust (strict)"("Visible"=FALSE) -> ()  [unwired: 2 in, 2 out]
            n143 = property on="Rev/Fwd" class="Clust (strict)"("Visible"=FALSE) -> ()  [unwired: 2 in, 2 out]
            n144 = case shown="\"White Balance  **\"" w238 {
              tunnel: w237 -> [w244 w253 w262 w271 w280 _ w286]
              tunnel: w236 -> [w242 w250 w259 w268 w277 _ _]
              frame "Size  **" {
                n145 = Index Array(array=w242) -> (element=w241:cluster{string[]})  [unwired: 1 in]
                n146 = call <vilib>:"NT Read String.vi"("Name"=w244) -> ("String"=w243:string)  [unwired: 9 in, 1 out]
                n147 = Unbundle(w241) -> (w239:string[])
                n148 = Match First String(2:w239, 3:w243) -> (0:w240:i32)  [unwired: 1 out]
                n149 = property on="Test Ring" class="Ring (strict)"("Value"=w240, "Strings []"=w239) -> ()  [unwired: 2 in, 2 out]
                n150 = property on="Test Ring" class="Ring (strict)"("Visible"=TRUE) -> ()  [unwired: 2 in, 2 out]
                n151 = property on="Test Slider" class="Slide (strict)"("Visible"=FALSE) -> ()  [unwired: 2 in, 2 out]
              }
              frame "White Balance  **" {
                n152 = Index Array(array=w250, index=1) -> (element=w251:cluster{string[]})
                n153 = call <vilib>:"NT Read String.vi"("Name"=w253) -> ("String"=w252:string)  [unwired: 9 in, 1 out]
                n154 = Unbundle(w251) -> (w248:string[])
                n155 = Match First String(2:w248, 3:w252) -> (0:w247:i32)  [unwired: 1 out]
                n156 = property on="Test Ring" class="Ring (strict)"("Value"=w247, "Strings []"=w248) -> ()  [unwired: 2 in, 2 out]
                n157 = property on="Test Ring" class="Ring (strict)"("Visible"=TRUE) -> ()  [unwired: 2 in, 2 out]
                n158 = property on="Test Slider" class="Slide (strict)"("Visible"=FALSE) -> ()  [unwired: 2 in, 2 out]
              }
              frame "Exposure  **" {
                n159 = Index Array(array=w259, index=2) -> (element=w260:cluster{string[]})
                n160 = call <vilib>:"NT Read String.vi"("Name"=w262) -> ("String"=w261:string)  [unwired: 9 in, 1 out]
                n161 = Unbundle(w260) -> (w256:string[])
                n162 = Match First String(2:w256, 3:w261) -> (0:w257:i32)  [unwired: 1 out]
                n163 = property on="Test Ring" class="Ring (strict)"("Value"=w257, "Strings []"=w256) -> ()  [unwired: 2 in, 2 out]
                n164 = property on="Test Ring" class="Ring (strict)"("Visible"=TRUE) -> ()  [unwired: 2 in, 2 out]
                n165 = property on="Test Slider" class="Slide (strict)"("Visible"=FALSE) -> ()  [unwired: 2 in, 2 out]
              }
              frame "Exposure Priority  **" {
                n166 = Index Array(array=w268, index=3) -> (element=w269:cluster{string[]})
                n167 = call <vilib>:"NT Read String.vi"("Name"=w271) -> ("String"=w270:string)  [unwired: 9 in, 1 out]
                n168 = Unbundle(w269) -> (w265:string[])
                n169 = Match First String(2:w265, 3:w270) -> (0:w266:i32)  [unwired: 1 out]
                n170 = property on="Test Ring" class="Ring (strict)"("Value"=w266, "Strings []"=w265) -> ()  [unwired: 2 in, 2 out]
                n171 = property on="Test Ring" class="Ring (strict)"("Visible"=TRUE) -> ()  [unwired: 2 in, 2 out]
                n172 = property on="Test Slider" class="Slide (strict)"("Visible"=FALSE) -> ()  [unwired: 2 in, 2 out]
              }
              frame "Color Enable  **" {
                n173 = Index Array(array=w277, index=4) -> (element=w278:cluster{string[]})
                n174 = call <vilib>:"NT Read String.vi"("Name"=w280) -> ("String"=w279:string)  [unwired: 9 in, 1 out]
                n175 = Unbundle(w278) -> (w274:string[])
                n176 = Match First String(2:w274, 3:w279) -> (0:w275:i32)  [unwired: 1 out]
                n177 = property on="Test Ring" class="Ring (strict)"("Value"=w275, "Strings []"=w274) -> ()  [unwired: 2 in, 2 out]
                n178 = property on="Test Ring" class="Ring (strict)"("Visible"=TRUE) -> ()  [unwired: 2 in, 2 out]
                n179 = property on="Test Slider" class="Slide (strict)"("Visible"=FALSE) -> ()  [unwired: 2 in, 2 out]
              }
              frame Default {
                n180 = property on="Test Ring" class="Ring (strict)"("Visible"=FALSE) -> ()  [unwired: 2 in, 2 out]
                n181 = property on="Test Slider" class="Slide (strict)"("Visible"=FALSE) -> ()  [unwired: 2 in, 2 out]
              }
              frame "Brightness  **", "Color Level  **", "Compression  **", "FPS  **", "Sharpness  **" {
                n182 = call <vilib>:"NT Read Number.vi"("Name"=w286) -> ("Numeric"=w285:dbl)  [unwired: 9 in, 1 out]
                n183 = local write "Test Slider"(w285) -> ()
                n184 = property on="Test Slider" class="Slide (strict)"("Visible"=TRUE, "Scale.Maximum"=100.0 ("Scale.Range:Maximum")) -> ()  [unwired: 2 in, 2 out]
                n185 = property on="Test Ring" class="Ring (strict)"("Visible"=FALSE) -> ()  [unwired: 2 in, 2 out]
              }
            }
          }
        }
        n186 = property on="Progress" class="Clust (strict)"("Visible"=FALSE) -> ()  [unwired: 2 in, 2 out]
      }
      event "Test Name": Mouse Enter {
        # "Populate the ring with the list of tests"
        n187 = event-data() -> ()  [unwired: 1 in, 1 out]
        n188 = call <vilib>:"NT Read String Array.vi"("Name"="TestMode/TestList") -> ("String Array"=w294:string[])  [unwired: 9 in, 1 out]
        n189 = Build Array (concatenate)("Select the test to run...", w294) -> (w293:string[])
        n190 = property on="Test Name" class="Ring (strict)"("Strings []"=w293) -> ()  [unwired: 2 in, 2 out]
      }
      event "Test Name": Value Change {
        w296 = FALSE ("Visible")
        # "Tell the robot the test name to run"
        n191 = event-data() -> ("NewVal"=w300:u16)  [unwired: 1 in]
        n192 = property on="Test Name" class="Ring (strict)"() -> ("Strings []"=w301:string[])  [unwired: 2 in, 2 out]
        n193 = local write "Progress"(T7 {"Test Progress"=0, "Test Progress Text"=""} ("Progress")) -> ()
        n194 = Index Array(array=w301, index=w300) -> (element=w299:string)
        n195 = call <vilib>:"NT Write String.vi"("String"=w299, "Name"="TestMode/TestName") -> ()  [unwired: 9 in, 1 out]
        n196 = property on="Progress" class="Clust (strict)"("Visible"=TRUE) -> ()  [unwired: 2 in, 2 out]
        n197 = property on="Motor" class="Clust (strict)"("Visible"=w296) -> ()  [unwired: 2 in, 2 out]
        n198 = property on="Test Slider" class="Slide (strict)"("Visible"=w296) -> ()  [unwired: 2 in, 2 out]
        n199 = property on="On/Off" class="Bool (strict)"("Visible"=w296) -> ()  [unwired: 2 in, 2 out]
        n200 = property on="Rev/Fwd" class="Clust (strict)"("Visible"=w296) -> ()  [unwired: 2 in, 2 out]
        n201 = property on="Test Ring" class="Ring (strict)"("Visible"=w296) -> ()  [unwired: 2 in, 2 out]
      }
      event "Listbox": Double Click {
        # "Shift clears all"
        # "Update symbols on the listbox"
        n202 = event-data() -> ("PlatMods.Shift"=w304:bool, "Row"=w306:i32)  [unwired: 1 in]
        n203 = case shown="True" w304 {
          tunnel: w306 -> [w310 _]
          tunnel: 1 -> [w309 _]
          frame False {
            n204 = property on="Listbox" class="LstBox (strict)"() -> ("Item Symbols"=w308:i32[])  [unwired: 2 in, 2 out]
            n205 = Replace Array Subset(array=w308, new element=w309, index=w310) -> (w307:i32[])
            n206 = property on="Listbox" class="LstBox (strict)"("Item Symbols"=w307) -> ()  [unwired: 2 in, 2 out]
          }
          frame True {
            w311 = 0 ("Top Row")
            n207 = property on="Listbox" class="LstBox (strict)"() -> ("Number of Rows"=w313:u32)  [unwired: 2 in, 2 out]
            n208 = Initialize Array(0, w313) -> (w312:i32[])
            n209 = property on="Listbox" class="LstBox (strict)"("Top Row"=w311, "Value"=w311, "Item Symbols"=w312) -> ()  [unwired: 2 in, 2 out]
          }
        }
      }
      event "Listbox": Key Down {
        # "Update symbols on the listbox\nLeft and right keys check and uncheck"
        n210 = event-data() -> ("VKey"=w317:T21)  [unwired: 1 in]
        n211 = case shown="\"Left\", \"Right\"" w317 {
          selector: w317 -> [w322 _]
          tunnel: eventvkey."Left" ("VKey") -> [w320 _]
          frame "Left", "Right" {
            n212 = Equal?(x=w320, y=w322) -> (x = y?=w321:bool)
            n213 = Select(t=0, s=w321, f=1) -> (s? t:f=w323:i32)
            n214 = property on="Listbox" class="LstBox (strict)"() -> ("Item Symbols"=w326:i32[])  [unwired: 2 in, 2 out]
            n215 = Replace Array Subset(array=w326, new element=w323, index="Listbox") -> (w325:i32[])
            n216 = property on="Listbox" class="LstBox (strict)"("Item Symbols"=w325) -> ()  [unwired: 2 in, 2 out]
          }
          frame Default {
          }
        }
      }
      event "DB Camera Config": Value Change {
        # "Show or hide the cluster of controls, store in ini file"
        n217 = event-data() -> ("NewVal"=w330:bool)  [unwired: 1 in]
        n218 = case shown="False" w330 {
          tunnel: w329 -> [w339 _]
          tunnel: [w332 w350] -> w328
          tunnel: w327 -> [w331 w350]
          frame False {
            w346 = "Camera"
            w349 = FALSE ("Visible")
            n219 = local read "Camera Settings"() -> (w338:T2)
            n220 = Index Array(array=w339) -> (element=w342:cluster{string[]})  [unwired: 1 in]
            n221 = Unbundle(w338) -> ("Frame Rate"=w337:i32, "Compression"=w336:i32, "Size"=w340:u16)
            n222 = Unbundle(w342) -> (w341:string[])
            n223 = Index Array(array=w341, index=w340) -> (element=w335:string)
            n224 = call-poly <vilib>:"Write Key.vi"("section"=w346, "value"=w335, "key"="Size", "refnum"=w331) -> ("refnum out"=w348:T19)  [unwired: 2 in, 5 out]
            n225 = call-poly <vilib>:"Write Key.vi"("section"=w346, "value"=w337, "key"="FrameRate", "refnum"=w348) -> ("refnum out"=w347:T19)  [unwired: 1 in, 6 out]
            n226 = property on="Camera Settings" class="Clust (strict)"("Visible"=w349) -> ()  [unwired: 2 in, 2 out]
            n227 = local write "DB Camera Config"(w349) -> ()
            n228 = call-poly <vilib>:"Write Key.vi"("section"=w346, "value"=w336, "key"="Compression", "refnum"=w347) -> ("refnum out"=w333:T19)  [unwired: 1 in, 6 out]
            n229 = call <vilib>:"Close Config Data.vi"("refnum"=w333) -> ("file path"=w334:path)  [unwired: 2 in, 8 out]
            n230 = call <vilib>:"Open Config Data.vi"("configuration file path"=w334) -> ("refnum"=w332:T19)  [unwired: 8 in, 2 out]
          }
          frame True {
            n231 = property on="Camera Settings" class="Clust (strict)"("Visible"=TRUE) -> ()  [unwired: 2 in, 2 out]
          }
        }
      }
      event "Camera Settings": Value Change {
        # "Update summary string when any elements of DB camera change"
        n232 = event-data() -> ("NewVal"=w363:T2)  [unwired: 1 in]
        n233 = Index Array(array=w359) -> (element=w358:cluster{string[]})  [unwired: 1 in]
        n234 = Unbundle(w363) -> ("Frame Rate"=w354:i32, "Compression"=w353:i32, "Size"=w356:u16)
        n235 = Unbundle(w358) -> (w357:string[])
        n236 = Index Array(array=w357, index=w356) -> (element=w355:string)
        n237 = Format Into String(format string="%s   %dfps   %d%%", w355, w354, w353) -> (resulting string=w360:string)  [unwired: 2 in, 1 out]
        n238 = Build Array(w360) -> (w361:string[])
        n239 = property on="DB Camera Config" class="Bool (strict)"("Strings [4]"=w361) -> ()  [unwired: 2 in, 2 out]
      }
      event "Motor.Enable": Value Change {
        # "When the test mode otor enable helper is set, update that\ntree row item's value"
        n240 = event-data() -> ("NewVal"=w369:bool)  [unwired: 1 in]
        n241 = Unbundle("Motor") -> ("Value"=w368:dbl)  [unwired: 1 out]
        n242 = Select(t=w368, s=w369, f=0.0) -> (s? t:f=w366:dbl)
        n243 = call <vilib>:"NT Write Number.vi"("Numeric"=w366, "Name"=w365) -> ()  [unwired: 9 in, 1 out]
      }
      event "Test Slider": Value Change {
        # "When the test mode slider helper is set, update that\ntree row item's value"
        n244 = event-data() -> ("NewVal"=w372:dbl)  [unwired: 1 in]
        n245 = call <vilib>:"NT Write Number.vi"("Numeric"=w372, "Name"=w373) -> ()  [unwired: 9 in, 1 out]
      }
      event "On/Off": Value Change {
        # "When the test mode on/off helper value is set, update that\ntree row item's value"
        n246 = event-data() -> ("NewVal"=w377:bool)  [unwired: 1 in]
        n247 = Boolean To (0,1)(Boolean=w377) -> (0, 1=w376:i16)
        n248 = call <vilib>:"NT Write Number.vi"("Numeric"=w376, "Name"=w375) -> ()  [unwired: 9 in, 1 out]
      }
      event "Rev/Fwd": Value Change {
        # "When the test mode helper value for relays is set, update that\ntree row item's value"
        n249 = event-data() -> ("NewVal.Forward"=w385:bool, "NewVal.Reverse"=w384:bool)  [unwired: 1 in]
        n250 = Boolean To (0,1)(Boolean=w385) -> (0, 1=w381:i16)
        n251 = Boolean To (0,1)(Boolean=w384) -> (0, 1=w383:i16)
        n252 = Negate(x=w383) -> (-x=w382:i16)
        n253 = Add(x=w381, y=w382) -> (x+y=w380:i16)
        n254 = call <vilib>:"NT Write Number.vi"("Numeric"=w380, "Name"=w379) -> ()  [unwired: 9 in, 1 out]
      }
      event "Test Ring": Value Change {
        # "When a test mode helper value is selected from the ring,\nset the tree item's variable to the string value"
        n255 = event-data() -> ("NewVal"=w389:u16)  [unwired: 1 in]
        n256 = property on="Test Ring" class="Ring (strict)"() -> ("Strings []"=w390:string[])  [unwired: 2 in, 2 out]
        n257 = Index Array(array=w390, index=w389) -> (element=w388:string)
        n258 = call <vilib>:"NT Write String.vi"("String"=w388, "Name"=w387) -> ()  [unwired: 9 in, 1 out]
      }
      event "Rec Mode": Value Change {
        # "Update globals for recording mode and path to read log from.\nClear when logging and let NetworkTables set path for vision to\nuse."
        n259 = event-data() -> ("NewVal"=w400:enum32{"Stop", "Record", "Playback"})  [unwired: 1 in]
        n260 = global write "WPI_DashboardLogging Global.vi" "Logging Filename"(path "") -> ()
        n261 = case shown="\"Playback\"" w400 {
          tunnel: w399 -> [_ w402 w410]
          tunnel: [_ _ w409] -> w396
          tunnel: [_ _ w408] -> _
          tunnel: w394 -> [_ _ w406]
          tunnel: cluster{i32, i32} {-250, 170} -> [_ _ w405]
          tunnel: [_ _ T22 {"Image Size"=TRUE, "Image Type"=TRUE, "Pixel Value"=TRUE, "ROI Information"=TRUE, "Zoom Factor"=FALSE} ("Image Information Shown:All Elements")] -> w392
          tunnel: [_ _ TRUE ("Zoom Factor")] -> w391
          frame Default {
          }
          frame "Stop", "Record" {
            # "Place Window too"
            n262 = invoke class="VI" method="FP.Close"(reference=w402) -> (reference out=w401:refnum<vi>)  [unwired: 2 in, 2 out]
            n263 = invoke class="VI" method="Abort VI"(reference=w401) -> ()  [unwired: 2 in, 3 out]
          }
          frame "Playback" {
            n264 = call "Open Playback Panel.vi"("Offset"=w405, "DB VI Ref"=w406, "Playback in"=w410) -> ("Playback out"=w407:refnum<vi>)  [unwired: 8 in]
            n265 = register-events(w407) -> (reference out=w409:refnum<event-registration>, error out=w408:errorcluster)  [unwired: 2 in]
          }
        }
        n266 = global write "WPI_DashboardLogging Global.vi" "Recording"(w400) -> ()
        n267 = property on="Camera Image" class="ImageControl"("Image Information Shown"=w392, "Image Information Visible"=w391) -> ()  [unwired: 2 in, 2 out]
        n268 = call <vilib>:"WPI_DashboardNT Log FieldName Cache.vi"("Operation"=enum16{"Lookup/Add", "Index", "Clear"}."Clear") -> ()  [unwired: 8 in, 3 out]
      }
      event Panel Close {
        w411 = enum32{"Stop", "Record", "Playback"}."Stop" ("Rec Mode")
        # "Playback window has been closed, abort"
        n269 = event-data() -> ()  [unwired: 1 in, 4 out]
        n270 = local write "Rec Mode"(w411) -> ()
        n271 = global write "WPI_DashboardLogging Global.vi" "Recording"(w411) -> ()
      }
      event Panel Close? {
        # "Abort playback window and ourself\nunless in development mode"
        n272 = event-data() -> ()  [unwired: 1 in, 4 out]
        n273 = invoke class="VI" method="FP.Close"(reference=w419) -> (reference out=w418:refnum<vi>)  [unwired: 2 in, 2 out]
        n274 = invoke class="VI" method="FP.Close"(reference=w413) -> (reference out=w414:refnum<vi>)  [unwired: 2 in, 2 out]
        n275 = invoke class="VI" method="Abort VI"(reference=w418) -> (error out=w417:errorcluster)  [unwired: 2 in, 2 out]
        n276 = disable-structure shown="RUN_TIME_ENGINE==False" {
          disable-tunnel: w417 -> [w420 _]
          disable-tunnel: [_ TRUE] -> w415
          frame condition #0 {
            n277 = invoke class="VI" method="Abort VI"(error in=w420) -> ()  [unwired: 2 in, 3 out]
          }
          frame condition #1 (active) {
            n278 = invoke class="VI" method="Abort VI"() -> ()  [unwired: 3 in, 3 out]
          }
        }
        n279 = invoke class="VI" method="Abort VI"(reference=w414) -> ()  [unwired: 2 in, 3 out]
        n280 = event-data("Discard?"=w415) -> ()  [unwired: 1 in, 1 out]
      }
      event "Vision": Value Change {
        # "Enable/Disable Compression slider.\nHW USB is hard-coded into the camera"
        n281 = event-data() -> ("NewVal"=w427:u16)  [unwired: 1 in]
        n282 = Equal?(x=w427, y=u32 2 ("milliseconds to wait")) -> (x = y?=w425:bool)
        n283 = Select(t=T23."Disabled and Grayed Out" ("Disabled"), s=w425, f=T23."Enabled" ("Disabled")) -> (s? t:f=w422:T23)
        n284 = property on="Compression" class="Slide (strict)"("DisabledEnum"=w422) -> ()  [unwired: 2 in, 2 out]
      }
      event "Auton List": Value Change {
        n285 = event-data() -> ()  [unwired: 1 in, 1 out]
        n286 = disable-structure shown="Disabled" {
          frame Disabled {
            n287 = case shown="True" FALSE {
              tunnel: _ -> [_ w456]
              frame False {
              }
              frame True {
                n288 = Current VI's Path() -> (path=w455:path)
                n289 = property on="Auton List" class="CmbBox"() -> ("Strings []"=w457)  [unwired: 2 in, 2 out]
                n290 = Strip Path(path=w455) -> (stripped path=w454:path)  [unwired: 1 out]
                n291 = disable-structure shown="RUN_TIME_ENGINE==True" {
                  disable-tunnel: [w458 w459] -> w450
                  disable-tunnel: w454 -> [w458 w460]
                  frame condition #0 (active) {
                  }
                  frame condition #1 {
                    n292 = Strip Path(path=w460) -> (stripped path=w459:path)  [unwired: 1 out]
                  }
                }
                n293 = Index Array(array=w457, index=w456) -> (element=w433)
                n294 = call-poly <vilib>:"Set Cursor.vi"("icon"=u16 2) -> ("error out"=w437:errorcluster)  [unwired: 9 in, 1 out]
                n295 = Concatenate Strings(w433, ".txt" ("string")) -> (w431:string)
                n296 = Build Path(base path=w450, name or relative path="Scripts") -> (appended path=w446:path)
                n297 = Build Path(base path=w450, name or relative path="Tools") -> (appended path=w448:path)
                n298 = Build Path(base path=w446, name or relative path=w431) -> (appended path=w445:path)
                n299 = Format Into String(format string="%s\\\\pscp -pw \"\" \"admin@roboRIO-3005.local:/home/lvuser/natinst/LabVIEW Data/Scripts/%s.*\" \"%s\"", error in=w437, w448, w433, w445) -> (resulting string=w452:string)  [unwired: 1 in, 1 out]
                "CMD" <- w452
                n300 = call <vilib>:"System Exec.vi"("run minimized? (F)"=TRUE, "command line"=w452) -> ("error out"=w436:errorcluster)  [unwired: 6 in, 3 out]
                n301 = property on="Auton Edit Area" class="Str"("DisabledEnum"=T23."Disabled" ("Disabled")) -> ()  [unwired: 2 in, 2 out]
                n302 = call-poly <vilib>:"Set Cursor.vi"("error in (no error)"=w436) -> ("error out"=w434:errorcluster)  [unwired: 9 in, 1 out]
                n303 = Open/Create/Replace File(file path (use dialog)=w445, error in=w434) -> (refnum out=w444:refnum<file>, error out=w443:errorcluster)  [unwired: 4 in, 1 out]
                n304 = Read from Text File(file (use dialog)=w444, error in=w443) -> (refnum out=w442:refnum<file>, text=w440:string, error out=w441:errorcluster)  [unwired: 2 in, 1 out]
                n305 = local write "Auton Edit Area"(w440) -> ()
                n306 = Close File(refnum=w442, error in=w441) -> (path=→"path":path)  [unwired: 1 out]
              }
            }
          }
          frame Enabled {
          }
        }
      }
      event "Enable Scripting": Value Change {
        n307 = event-data() -> ()  [unwired: 1 in, 6 out]
        n308 = property on="Auton List" class="CmbBox"() -> ("Value"=w461:string)  [unwired: 2 in, 2 out]
        n309 = property on="Auton List" class="CmbBox"("Val(Sgnl)"=w461) -> ()  [unwired: 2 in, 2 out]
      }
      event "Save": Value Change {
        n310 = event-data() -> ()  [unwired: 1 in, 1 out]
        n311 = Current VI's Path() -> (path=w485:path)
        n312 = local read "path"() -> (w472:path)
        n313 = Strip Path(path=w485) -> (stripped path=w484:path)  [unwired: 1 out]
        n314 = Open/Create/Replace File(file path (use dialog)=w472, operation (0:open)=T24."replace") -> (refnum out=w470:refnum<file>, error out=w469:errorcluster)  [unwired: 4 in, 1 out]
        n315 = disable-structure shown="RUN_TIME_ENGINE==True" {
          disable-tunnel: [w487 w488] -> w480
          disable-tunnel: w484 -> [w487 w489]
          frame condition #0 (active) {
          }
          frame condition #1 {
            n316 = Strip Path(path=w489) -> (stripped path=w488:path)  [unwired: 1 out]
          }
        }
        n317 = Write to Text File(file (use dialog)=w470, text="Auton Edit Area", error in=w469) -> (refnum out=w468:refnum<file>, error out=w467:errorcluster)  [unwired: 1 in, 1 out]
        n318 = call-poly <vilib>:"Set Cursor.vi"("icon"=u16 2) -> ("error out"=w475:errorcluster)  [unwired: 9 in, 1 out]
        n319 = Close File(refnum=w468, error in=w467) -> (path=w466:path)  [unwired: 1 out]
        n320 = Build Path(base path=w480, name or relative path="Tools") -> (appended path=w478:path)
        n321 = Strip Path(path=w466) -> (name=w473:string)  [unwired: 1 out]
        n322 = Format Into String(format string="%s\\\\pscp -pw \"\" \"%s\" \"admin@roboRIO-3005.local:/home/lvuser/natinst/LabVIEW Data/Scripts/%s\" ", error in=w475, w478, w466, w473) -> (resulting string=w482:string)  [unwired: 1 in, 1 out]
        n323 = call <vilib>:"System Exec.vi"("run minimized? (F)"=TRUE, "command line"=w482) -> ("error out"=w474:errorcluster, "standard error"=w464:string, "standard output"=w463:string)  [unwired: 6 in, 1 out]
        n324 = property on="Auton Edit Area" class="Str"("DisabledEnum"=T23."Disabled" ("Disabled")) -> ()  [unwired: 2 in, 2 out]
        n325 = call-poly <vilib>:"Set Cursor.vi"("error in (no error)"=w474) -> ()  [unwired: 9 in, 2 out]
      }
      event "Edit": Value Change {
        n326 = event-data() -> ("NewVal"=w490:bool)  [unwired: 1 in]
        n327 = case shown="True" w490 {
          tunnel: [TRUE ("Visible") FALSE ("Visible")] -> w493
          tunnel: [T23."Enabled" ("Disabled") T23."Disabled" ("Disabled")] -> w491
          frame True {
          }
          frame False {
          }
        }
        n328 = property on="Save" class="Bool"("Visible"=w493) -> ()  [unwired: 2 in, 2 out]
        n329 = property on="Auton Edit Area" class="Str"("DisabledEnum"=w491) -> ()  [unwired: 2 in, 2 out]
      }
    }
  }
  n330 = while {
    tunnel: w41 -> [w499]
    i -> [w502]
    stop <- FALSE stop-if-true
    n331 = Wait (ms)(milliseconds to wait=u32 100) -> ()  [unwired: 1 out]
    n332 = case shown="\"Stop\", Default" "Rec Mode" {
      tunnel: w502 -> [_ _ w517]
      tunnel: [u32 2829099 ("Base Color") u32 11141120 ("Target Color") w506] -> w498
      frame "Stop", Default {
        # "Reset the color, extra updates don't cost much"
      }
      frame "Record" {
      }
      frame "Playback" {
        # "Playback"
        n333 = Quotient & Remainder(x=w517, y=u32 50 ("milliseconds to wait")) -> (x-y*floor(x/y)=w513:u32)  [unwired: 1 out]
        n334 = Divide(x=w513, y=u32 50 ("milliseconds to wait")) -> (x/y=w510:dbl)
        n335 = Multiply(x=6.283185307179586, y=w510) -> (x*y=w515:dbl)
        n336 = Sine(x=w515) -> (sin(x)=w514:dbl)
        n337 = Absolute Value(x=w514) -> (abs(x)=w507:dbl)
        n338 = call "Interpolate RGB Color.vi"("Proportion"=w507, "Target Color"=u32 30976, "Base Color"=u32 2829099) -> ("Result Color"=w506:u32)  [unwired: 8 in]
      }
    }
    n339 = property class="Pane"(reference=w499, "PaneColor"=w498) -> ()  [unwired: 1 in, 2 out]
  }
  n340 = TCP Create Listener(10:u16 1741 ("timeout ms (25000)")) -> (3:w4:refnum<k5>)  [unwired: 4 in, 2 out]
  n341 = while {
    tunnel: w4 -> [w519]
    stop <- FALSE stop-if-true
    n342 = TCP Wait On Listener(11:w519) -> (4:w518:refnum<k5>)  [unwired: 3 in, 4 out]
    n343 = local write "TCP"(w518) -> ()
  }
  n344 = property on="On/Off" class="Bool (strict)"("Visible"=w9) -> ()  [unwired: 2 in, 2 out]
  n345 = property on="Motor" class="Clust (strict)"("Visible"=w9) -> ()  [unwired: 2 in, 2 out]
  n346 = property on="Progress" class="Clust (strict)"("Visible"=w9) -> ()  [unwired: 2 in, 2 out]
  n347 = property on="Test Ring" class="Ring (strict)"("Visible"=w9) -> ()  [unwired: 2 in, 2 out]
  n348 = property on="Rev/Fwd" class="Clust (strict)"("Visible"=w9) -> ()  [unwired: 2 in, 2 out]
  n349 = property on="Camera Settings" class="Clust (strict)"("Visible"=w9) -> ()  [unwired: 2 in, 2 out]
  n350 = local write "DB Camera Config"(w9) -> ()
  n351 = global write "WPI_DashboardLogging Global.vi" "Recording"(w35) -> ()
  n352 = local write "Rec Mode"(w35) -> ()
